vi "Get Crossing Point.vi"(10 "Vector 2":refnum<class "Vector.lvclass">, 11 "Vector in":refnum<class "Vector.lvclass">) -> (2 "Coordinate":T1, 3 "In Future?":bool)   [LabVIEW 2021, in "Vector.lvclass"]
uses:
  Vector.lvclass
  High Res Arithmetic/Rational Number.lvclass
  Vector.lvclass/Vector.ctl
  Read p_x.vi
  Read p_y.vi
  Read v_x.vi
  Read v_y.vi
  Hi Res Arithm Test/Create.vi
panel:
  out "Coordinate 2":T1
  out "A":refnum<class "Rational Number.lvclass">
  out "B":refnum<class "Rational Number.lvclass">
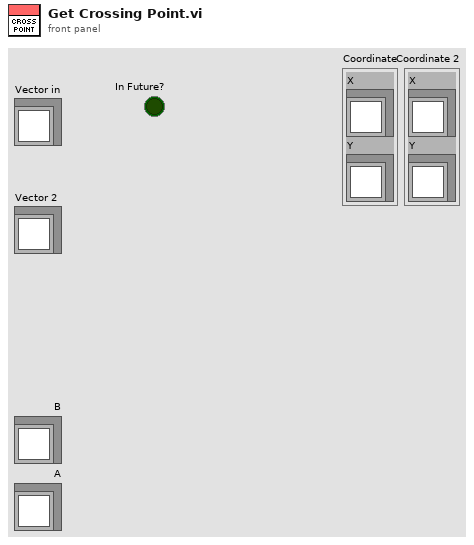
[diagram p1: front panel]
types:
  T1 = cluster{"X":refnum<class "Rational Number.lvclass">, "Y":refnum<class "Rational Number.lvclass">}
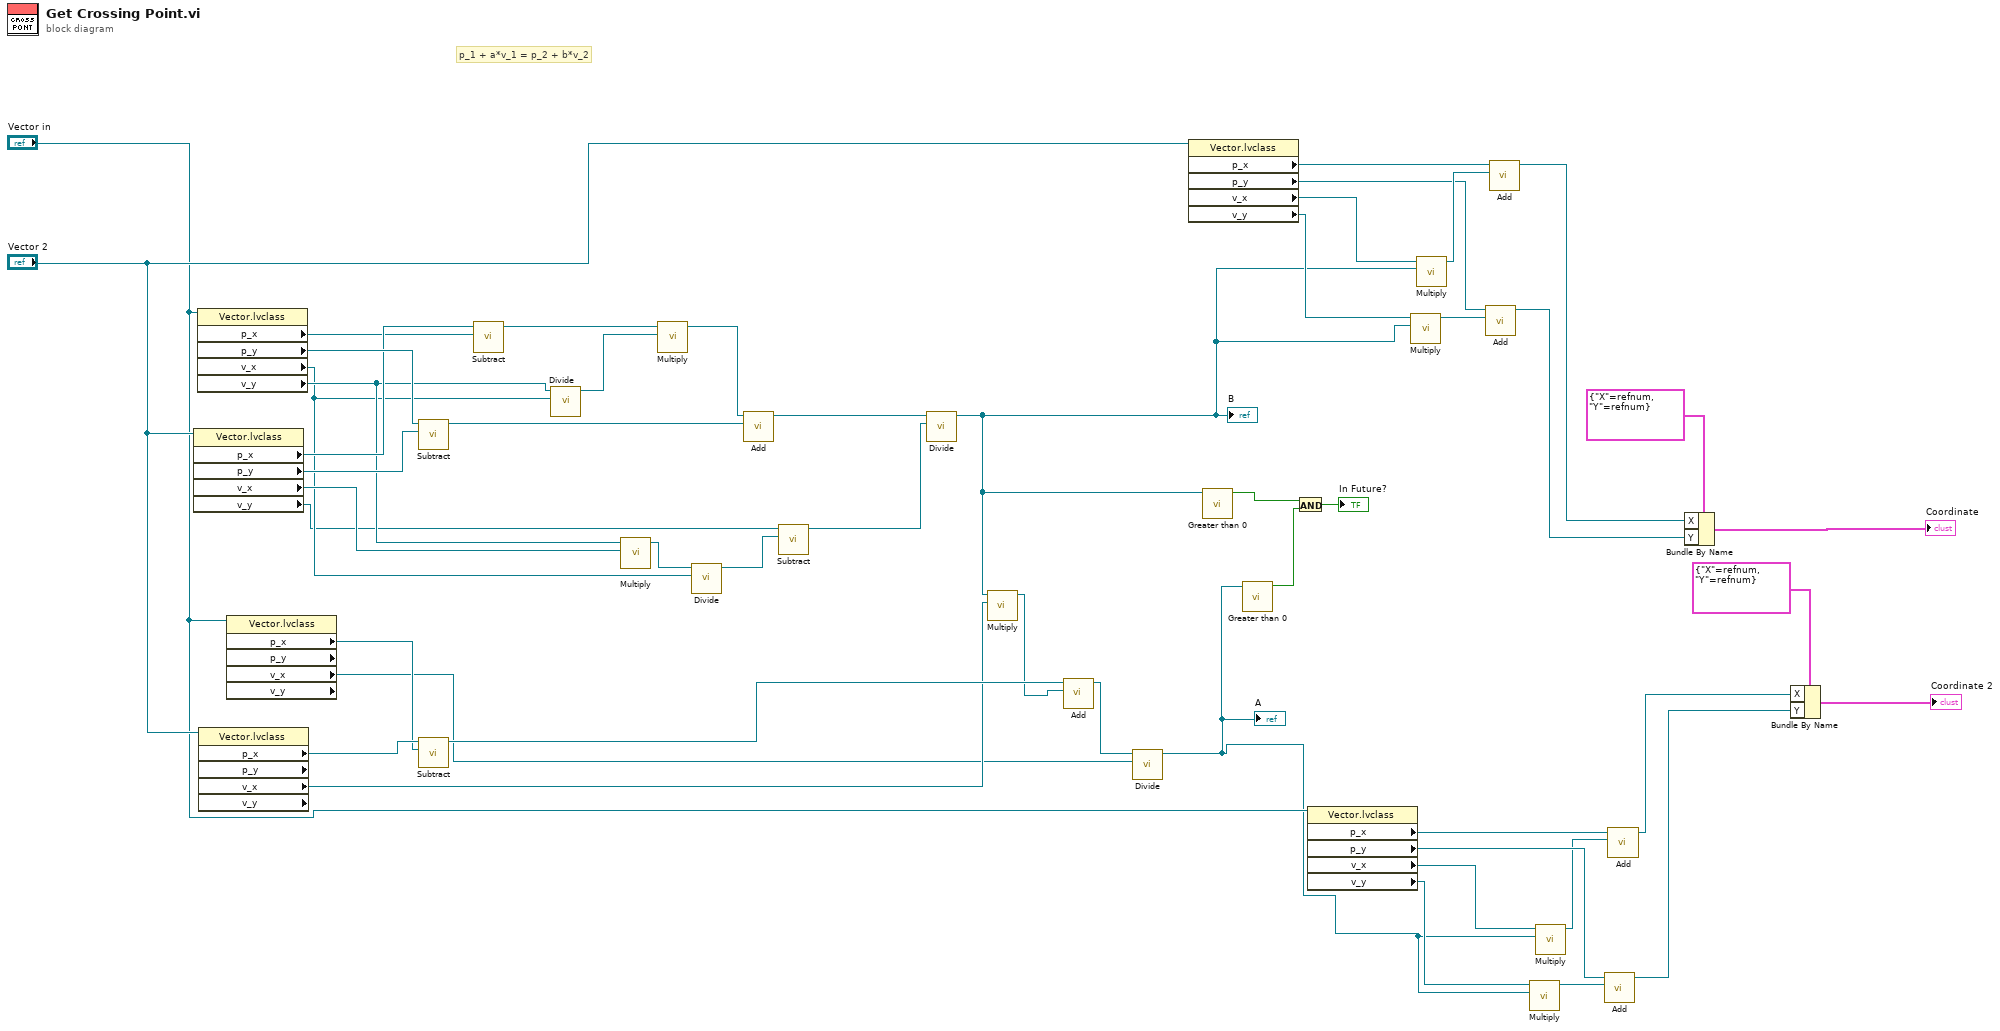
[diagram p0: block diagram]
diagram:
  # "p_1 + a*v_1 = p_2 + b*v_2"
  n1 = property class="Vector.lvclass"(reference="Vector 2") -> ("p_x"=w44:refnum<class "Rational Number.lvclass">, "p_y"=w45:refnum<class "Rational Number.lvclass">, "v_x"=w36:refnum<class "Rational Number.lvclass">, "v_y"=w32:refnum<class "Rational Number.lvclass">)  [unwired: 1 in, 2 out]
  n2 = property class="Vector.lvclass"(reference="Vector in") -> ("p_x"=w43:refnum<class "Rational Number.lvclass">, "p_y"=w46:refnum<class "Rational Number.lvclass">, "v_x"=w34:refnum<class "Rational Number.lvclass">, "v_y"=w37:refnum<class "Rational Number.lvclass">)  [unwired: 1 in, 2 out]
  n3 = property class="Vector.lvclass" props=["p_x", "p_y", "v_x", "v_y"](reference="Vector 2") -> ("p_x"=w18:refnum<class "Rational Number.lvclass">, "v_x"=w14:refnum<class "Rational Number.lvclass">)  [unwired: 1 in, 4 out]
  n4 = property class="Vector.lvclass" props=["p_x", "p_y", "v_x", "v_y"](reference="Vector in") -> ("p_x"=w17:refnum<class "Rational Number.lvclass">, "v_x"=w11:refnum<class "Rational Number.lvclass">)  [unwired: 1 in, 4 out]
  n5 = call "Subtract.vi"("High Res Arithmetic 2"=w45, "High Res Arithmetic 1"=w46) -> ("High Res Arithmetic sum"=w40:refnum<class "Rational Number.lvclass">)  [unwired: 8 in, 1 out]
  n6 = call "Subtract.vi"("High Res Arithmetic 2"=w17, "High Res Arithmetic 1"=w18) -> ("High Res Arithmetic sum"=w16:refnum<class "Rational Number.lvclass">)  [unwired: 8 in, 1 out]
  n7 = call "Subtract.vi"("High Res Arithmetic 2"=w43, "High Res Arithmetic 1"=w44) -> ("High Res Arithmetic sum"=w42:refnum<class "Rational Number.lvclass">)  [unwired: 8 in, 1 out]
  n8 = call "Divide.vi"("High Res Arithmetic 2"=w34, "High Res Arithmetic 1"=w37) -> ("High Res Arithmetic sum"=w41:refnum<class "Rational Number.lvclass">)  [unwired: 8 in, 1 out]
  n9 = call "Multiply.vi"("High Res Arithmetic 2"=w36, "High Res Arithmetic 1"=w37) -> ("High Res Arithmetic sum"=w35:refnum<class "Rational Number.lvclass">)  [unwired: 8 in, 1 out]
  n10 = call "Multiply.vi"("High Res Arithmetic 2"=w41, "High Res Arithmetic 1"=w42) -> ("High Res Arithmetic sum"=w39:refnum<class "Rational Number.lvclass">)  [unwired: 8 in, 1 out]
  n11 = call "Divide.vi"("High Res Arithmetic 2"=w34, "High Res Arithmetic 1"=w35) -> ("High Res Arithmetic sum"=w33:refnum<class "Rational Number.lvclass">)  [unwired: 8 in, 1 out]
  n12 = call "Add.vi"("High Res Arithmetic 2"=w40, "High Res Arithmetic 1"=w39) -> ("High Res Arithmetic sum"=w38:refnum<class "Rational Number.lvclass">)  [unwired: 8 in, 1 out]
  n13 = call "Subtract.vi"("High Res Arithmetic 2"=w33, "High Res Arithmetic 1"=w32) -> ("High Res Arithmetic sum"=w31:refnum<class "Rational Number.lvclass">)  [unwired: 8 in, 1 out]
  n14 = call "Divide.vi"("High Res Arithmetic 2"=w31, "High Res Arithmetic 1"=w38) -> ("High Res Arithmetic sum"=w15:refnum<class "Rational Number.lvclass">)  [unwired: 8 in, 1 out]
  "B" <- w15
  n15 = call "Multiply.vi"("High Res Arithmetic 2"=w14, "High Res Arithmetic 1"=w15) -> ("High Res Arithmetic sum"=w13:refnum<class "Rational Number.lvclass">)  [unwired: 8 in, 1 out]
  n16 = call "Add.vi"("High Res Arithmetic 2"=w13, "High Res Arithmetic 1"=w16) -> ("High Res Arithmetic sum"=w12:refnum<class "Rational Number.lvclass">)  [unwired: 8 in, 1 out]
  n17 = call "Divide.vi"("High Res Arithmetic 2"=w11, "High Res Arithmetic 1"=w12) -> ("High Res Arithmetic sum"=w1:refnum<class "Rational Number.lvclass">)  [unwired: 8 in, 1 out]
  "A" <- w1
  n18 = property class="Vector.lvclass"(reference="Vector 2") -> ("p_x"=w25:refnum<class "Rational Number.lvclass">, "p_y"=w22:refnum<class "Rational Number.lvclass">, "v_x"=w27:refnum<class "Rational Number.lvclass">, "v_y"=w26:refnum<class "Rational Number.lvclass">)  [unwired: 1 in, 2 out]
  n19 = call "Greater than 0.vi"("Rational Number in"=w15) -> ("Greater than 0?"=w30:bool)  [unwired: 10 in]
  n20 = call "Greater than 0.vi"("Rational Number in"=w1) -> ("Greater than 0?"=w29:bool)  [unwired: 10 in]
  n21 = And(x=w30, y=w29) -> (x .and. y?=→"In Future?":bool)
  n22 = property class="Vector.lvclass"(reference="Vector in") -> ("p_x"=w7:refnum<class "Rational Number.lvclass">, "p_y"=w10:refnum<class "Rational Number.lvclass">, "v_x"=w5:refnum<class "Rational Number.lvclass">, "v_y"=w6:refnum<class "Rational Number.lvclass">)  [unwired: 1 in, 2 out]
  n23 = call "Multiply.vi"("High Res Arithmetic 2"=w15, "High Res Arithmetic 1"=w26) -> ("High Res Arithmetic sum"=w23:refnum<class "Rational Number.lvclass">)  [unwired: 8 in, 1 out]
  n24 = call "Multiply.vi"("High Res Arithmetic 2"=w15, "High Res Arithmetic 1"=w27) -> ("High Res Arithmetic sum"=w24:refnum<class "Rational Number.lvclass">)  [unwired: 8 in, 1 out]
  n25 = call "Add.vi"("High Res Arithmetic 2"=w23, "High Res Arithmetic 1"=w22) -> ("High Res Arithmetic sum"=w19:refnum<class "Rational Number.lvclass">)  [unwired: 8 in, 1 out]
  n26 = call "Add.vi"("High Res Arithmetic 2"=w24, "High Res Arithmetic 1"=w25) -> ("High Res Arithmetic sum"=w20:refnum<class "Rational Number.lvclass">)  [unwired: 8 in, 1 out]
  n27 = call "Multiply.vi"("High Res Arithmetic 2"=w1, "High Res Arithmetic 1"=w6) -> ("High Res Arithmetic sum"=w9:refnum<class "Rational Number.lvclass">)  [unwired: 8 in, 1 out]
  n28 = call "Multiply.vi"("High Res Arithmetic 2"=w1, "High Res Arithmetic 1"=w5) -> ("High Res Arithmetic sum"=w8:refnum<class "Rational Number.lvclass">)  [unwired: 8 in, 1 out]
  n29 = call "Add.vi"("High Res Arithmetic 2"=w9, "High Res Arithmetic 1"=w10) -> ("High Res Arithmetic sum"=w2:refnum<class "Rational Number.lvclass">)  [unwired: 8 in, 1 out]
  n30 = call "Add.vi"("High Res Arithmetic 2"=w8, "High Res Arithmetic 1"=w7) -> ("High Res Arithmetic sum"=w3:refnum<class "Rational Number.lvclass">)  [unwired: 8 in, 1 out]
  n31 = Bundle By Name(cluster=T1 {"X"=refnum, "Y"=refnum} ("Coordinate"), "X"=w20, "Y"=w19) -> (→"Coordinate":T1)
  n32 = Bundle By Name(cluster=T1 {"X"=refnum, "Y"=refnum} ("Coordinate"), "X"=w3, "Y"=w2) -> (→"Coordinate 2":T1)
